vi "Read Config info.vi"(11 "AM-AM in":refnum<class "AM-AM.lvclass">) -> (2 "Config info":T1 {"Frequency"."Array" format="%#_6p"; "Power"."Array" format="%#_6p"}, 3 "AM-AM out":refnum<class "AM-AM.lvclass">)   [LabVIEW 2020, in "AM-AM.lvclass"]
uses:
  AM-AM.lvclass
  Controls/Config info.ctl
  Controls/Loop order.ctl
  AM-AM.lvclass/AM-AM.ctl
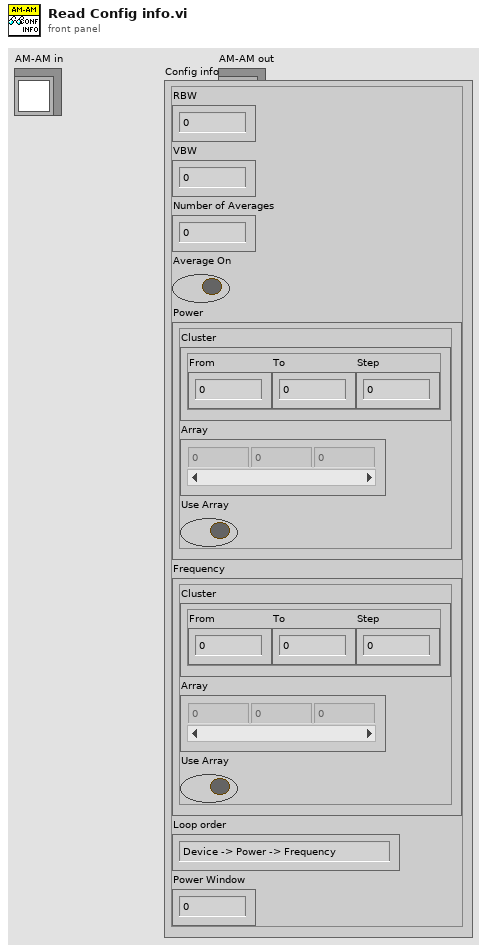
[diagram p1: front panel]
types:
  T1 = typedef "AM-AM.lvclass/Config info.ctl" = cluster{"RBW":dbl, "VBW ":dbl, "Number of Averages":dbl, "Average On":bool, "Power":cluster{"Cluster ":cluster{"From":dbl, "To":dbl, "Step":dbl}, "Array":dbl[], "Use Array":bool}, "Frequency":cluster{"Cluster ":cluster{"From":dbl, "To":dbl, "Step":dbl}, "Array":dbl[], "Use Array":bool}, "Loop order":T2, "Power Window":dbl}
  T2 = typedef "AM-AM.lvclass/Loop order.ctl" = enum16{"Device -> Power -> Frequency", "Device -> Frequency -> Power"}
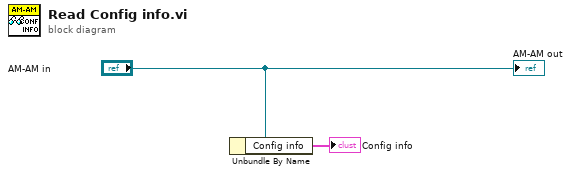
[diagram p0: block diagram]
diagram:
  n1 = Unbundle By Name("AM-AM in") -> ("Config info"=→"Config info":T1)
  "AM-AM out" <- "AM-AM in"
